vi "Clear.vi"(8 "error in (no error)":errorcluster, 11 "senseHatDisplay in":refnum<class "RPI.SenseHat.Display.lvclass">) -> (0 "error out":errorcluster, 3 "senseHatDisplay out":refnum<class "RPI.SenseHat.Display.lvclass">)   [LabVIEW 2020, in "RPI.SenseHat.Display.lvlib" / "RPI.SenseHat.Display.lvclass"]
doc: "Fills the screen with Black color.\n\nNote: Requires a call to Update to affect the physical screen."
uses:
  RPI.SenseHat.Display.lvclass
  Color/Color.lvclass
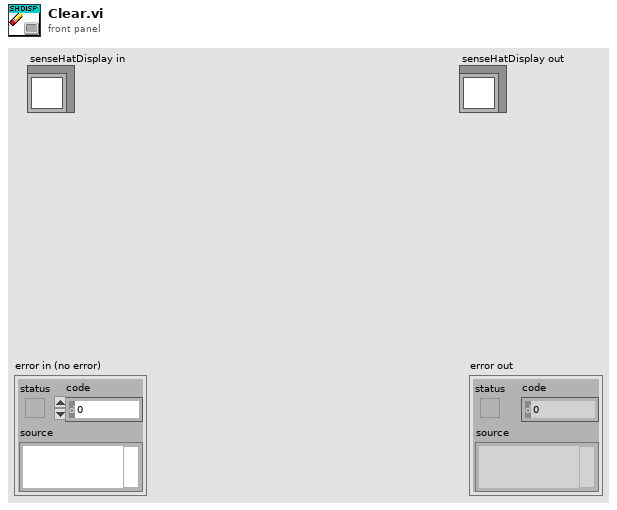
[diagram p1: front panel]
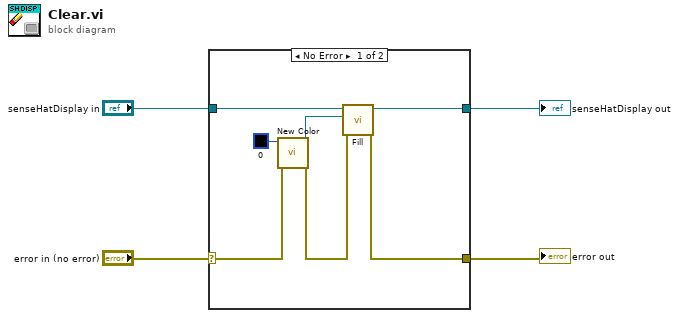
[diagram p0: block diagram]
diagram:
  n1 = case shown="No Error" "error in (no error)" {
    selector: "error in (no error)" -> [w8 w13]
    tunnel: [w6 w13] -> w3
    tunnel: [w10 w12] -> w1
    tunnel: "senseHatDisplay in" -> [w11 w12]
    frame No Error {
      n2 = call "New Color.vi"("error in (no error)"=w8, "Color Box"=u32 0) -> ("error out"=w7:errorcluster, "Color out"=w9:refnum<class "Color.lvclass">)  [unwired: 8 in]
      n3 = call "Fill.vi"("error in (no error)"=w7, "Color"=w9, "senseHatDisplay in"=w11) -> ("error out"=w6:errorcluster, "senseHatDisplay out"=w10:refnum<class "RPI.SenseHat.Display.lvclass">)  [unwired: 7 in]
    }
    frame Error {
    }
  }
  "error out" <- w3
  "senseHatDisplay out" <- w1
